vi "Write Startup Model-View Configuration.vi"(9 "Model":refnum<class "IModel.lvclass">, 10 "Startup View":refnum<class "IViewable.lvclass">, 11 "IController In":refnum<class "IController.lvclass">) -> (3 "IController Out":refnum<class "IController.lvclass">)   [LabVIEW 2015, in "IController.lvlib" / "IController.lvclass"]
uses:
  IController.lvclass
  IViewable/IViewable/IViewable.lvclass
  IModel/IModel/IModel.lvclass
  IController.lvclass/IController.ctl
  IViewManager/IViewManager Messages/Launch Nested Views Msg/Launch Nested Views Msg.lvclass/Launch Nested Views Msg.ctl
  IViewManager/IViewManager/IViewManager.lvclass/IViewManager.ctl
  IViewManager/IViewManager Messages/Launch Nested Views Msg/Launch Nested Views Msg.lvclass
  IViewManager/IViewManager/IViewManager.lvclass
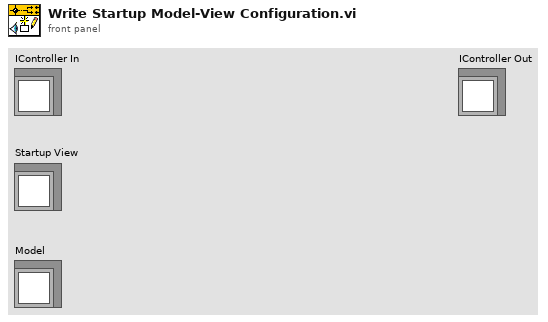
[diagram p1: front panel]
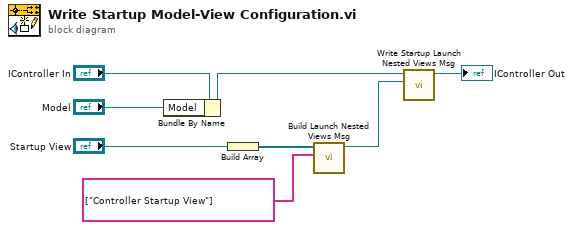
[diagram p0: block diagram]
diagram:
  n1 = Bundle By Name(cluster="IController In", "Model"="Model") -> (w2:refnum<class "IController.lvclass">)
  n2 = Build Array("Startup View") -> (w6:refnum<class "IViewable.lvclass">[])
  n3 = call "Build Launch Nested Views Msg.vi"("View Labels"=string[] ["Controller Startup View"] ("View Labels (optional)"), "Nested Views"=w6) -> ("Launch Nested Views Msg out"=w4:refnum<class "Launch Nested Views Msg.lvclass">)  [unwired: 8 in, 1 out]
  n4 = call "Write Startup Launch Nested Views Msg.vi"("Launch Nested Views Msg"=w4, "IViewManager in"=w2) -> ("IViewManager out"=→"IController Out":refnum<class "IController.lvclass">)  [unwired: 8 in, 1 out]
